vi "read_key_integer.vi"(7 "table":string, 8 "error in (no error)":errorcluster, 9 "default (0)":i64, 10 "key":string, 11 "toml in":refnum<class "toml.lvclass">) -> (0 "error out":errorcluster, 1 "value":i64, 3 "toml out":refnum<class "toml.lvclass">)   [LabVIEW 2020, in "toml.lvclass"]
uses:
  toml.lvclass
  toml.lvclass/toml.ctl
  Doc/Doc.lvclass
  Table/Table.lvclass
  Item/Item.lvclass
  Value/Value.lvclass
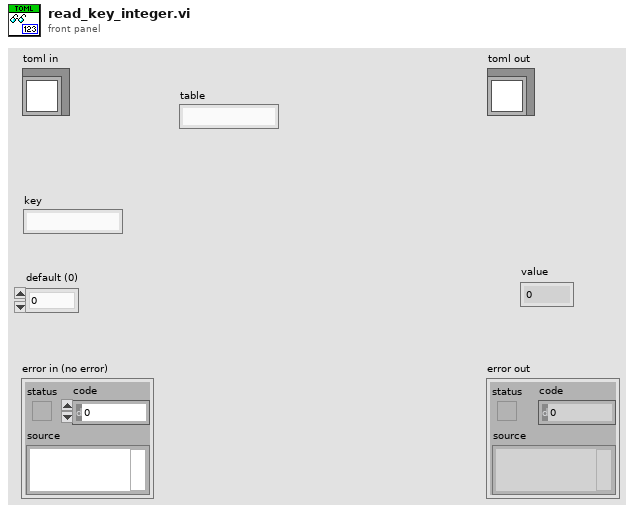
[diagram p1: front panel]
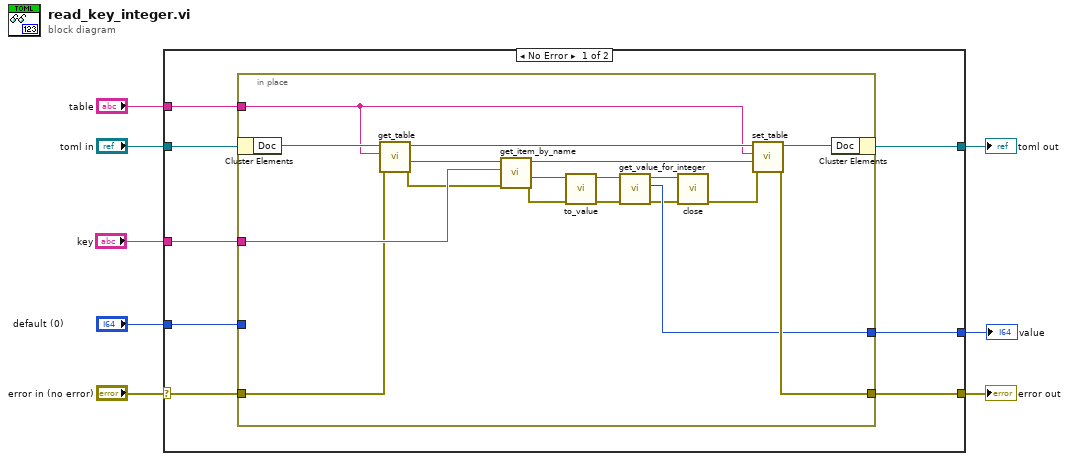
[diagram p0: block diagram]
diagram:
  n1 = case shown="No Error" "error in (no error)" {
    selector: "error in (no error)" -> [w10 w36]
    tunnel: [w11 w36] -> w7
    tunnel: [w15 w35] -> w5
    tunnel: "toml in" -> [w16 w35]
    tunnel: "table" -> [w14 _]
    tunnel: "key" -> [w13 _]
    tunnel: "default (0)" -> [w12 _]
    tunnel: [w9 _] -> w1
    frame No Error {
      n2 = in-place {
        in-place-border: w14 -> [w26]
        in-place-border: w13 -> [w29]
        in-place-border: w12 -> [_]
        in-place-border: [w28] -> w11
        in-place-border: w10 -> [w27]
        in-place-border: [w20] -> w9
        n3 = in-place-cluster #1(w16) -> ("Doc"=w31:refnum<class "Doc.lvclass">)
        n4 = call "get_table.vi"("error in (no error)"=w27, "table_name"=w26, "Doc in"=w31) -> ("error out"=w25:errorcluster, "Table"=w34:refnum<class "Table.lvclass">, "Doc out"=w33:refnum<class "Doc.lvclass">)  [unwired: 6 in]
        n5 = call "get_item_by_name.vi"("error in (no error)"=w25, "item_name"=w29, "Table in"=w34) -> ("error out"=w21:errorcluster, "Item"=w24:refnum<class "Item.lvclass">, "Table out"=w32:refnum<class "Table.lvclass">)  [unwired: 6 in]
        n6 = call "to_value.vi"("error in (no error)"=w21, "Item in"=w24) -> ("error out"=w22:errorcluster, "Value out"=w23:refnum<class "Value.lvclass">)  [unwired: 8 in]
        n7 = call "get_value_for_integer.vi"("error in (no error)"=w22, "Value in"=w23) -> ("error out"=w18:errorcluster, "integer_value"=w20:i64, "Value out"=w19:refnum<class "Value.lvclass">)  [unwired: 7 in]
        n8 = call "close.vi"("error in (no error)"=w18, "Value in"=w19) -> ("error out"=w17:errorcluster)  [unwired: 9 in]
        n9 = call "set_table.vi"("error in (no error)"=w17, "Table"=w32, "table_name"=w26, "Doc in"=w33) -> ("error out"=w28:errorcluster, "Doc out"=w30:refnum<class "Doc.lvclass">)  [unwired: 6 in]
        n10 = in-place-cluster #1("Doc"=w30) -> (w15:refnum<class "toml.lvclass">)
      }
    }
    frame Error {
    }
  }
  "error out" <- w7
  "toml out" <- w5
  "value" <- w1
